vi "LP MDrive_Home.vi"(0 "VISA IN":refnum<visa-resource-name>="COM1", 1 "Home Direction":string="1", 5 "error in":errorcluster, 6 "Max Velocity to Home":string="1500", 9 "Mdrive Mode":T1=enum."Party Mode", 11 "Device Name":string="R", 12 "Timeout":u32=30000) -> (14 "VISA OUT":refnum<visa-resource-name>="COM1", 15 "Moved":bool, 19 "error out":errorcluster)   [LabVIEW 2015]
uses:
  MCode_LV_86/MDrive Mode.ctl
  MCode_LV_86/Set Parameter.ctl
  Stream/LP Globals.vi
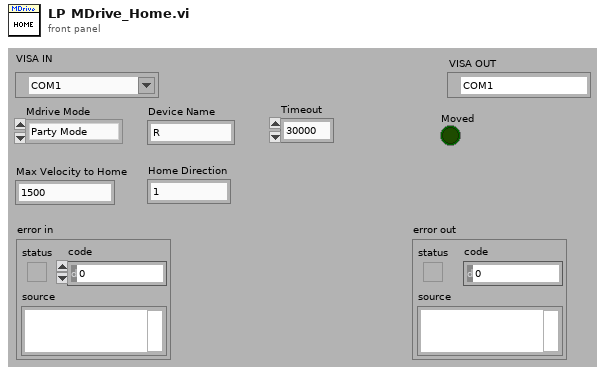
[diagram p1: front panel]
types:
  T1 = typedef "MDrive Mode.ctl" = enum16{"Normal Mode", "Party Mode"}
  T2 = typedef "Set Parameter.ctl" = enum16{"Acceleration (A)", "Baud Rate (BD)", "Counter 1 (C1)", "Counter 2 (C2)", "Control C Software Reset (CE)", "Check Sum Enable (CK)", "Clock Mode (CM)", "Clock Mode Ratio (CR)", "Clock Mode Out Step Width (CW)", "Deceleration (D)", "Digital Filtering, Input 1 (D1)", "Digital Filtering, Input 2 (D2)", "Digital Filtering, Input 3 (D3)", "Digital Filtering, Input 4 (D4)", "Digital Filtering, Input 5 (D5)", "Digital Filtering, Input 9 (D9)", "Digital Filtering, Input 10 (D10)", "Digital Filtering, Input 11 (D11)", "Digital Filtering, Input 12 (D12)", "Deadband (DB)", "Decrement Variable (DC)", "Enable/Disable Drive (DE)", "Device Name (DN)", "End Program Execution (E)", "Encoder Function Enable (EE)", "Encoder Lines (EL)", "Echo Mode (EM)", "Error Clear (ER)", "Escape (ES)", "Execute Program at Address (EX)", "Factory Default (FD)", "Hold (H)", "Hold Current (HC)", "Hold Current Encoder Index (HI)", "Home to Home Switch (HM)", "Home to Delay Time (HT)", "Increment Variable (IC)", "Initialize Parameters to NVM (IP)", "Input into Variable (IV)", "Jog Enable (JE)", "Limit Stop Mode (LM)", "Move Absolute (MA)", "Move Relative (MR)", "MicroStepping Select (MS)", "Motor Settling Delay Time (MT)", "Output 1 (O1)", "Output 2 (O2)", "Output 3 (O3)", "Output 4 (O4)", "Output 9 (O9)", "Output 10 (O10)", "Output 11 (O11)", "Output 12 (O12)", "Output High Byte (9-12) (OH)", "Output Low Byte (1-4) (OL)", "Output Total (1-4 and 9-12) (OT)", "Position (P)", "Position Maintenance (PM)", "Party Mode (PY)", "Register 1 (R1)", "Register 2 (R2)", "Register 3 (R3)", "Register 4 (R4)", "Run Current (RC)", "Stall Factor (SF)", "Slew (SL)", "Stall Mode Set (SM)", "Upgrade Firmware (UG)", "Velocity Initial (VI)", "Velocity Maximum (VM)", "Set Input #1 as Home (S1)", "Save (S)", "Save DN+PY (NameS)", "Active Party Mode (0x0A)", "Set Input #1 (S1) as Limit- Active Floating", "Set Input #2 (S2) as Limit+ Active Floating", "Set Input #1 as Home (S1) Active Floating", "Set Input #1 as Home (S2) Active Floating", "Set Input #1 (S1) as Limit+ Active Floating", "Set Input #2 (S2) as Limit- Active Floating", "Hybrid Mode (AS)"}
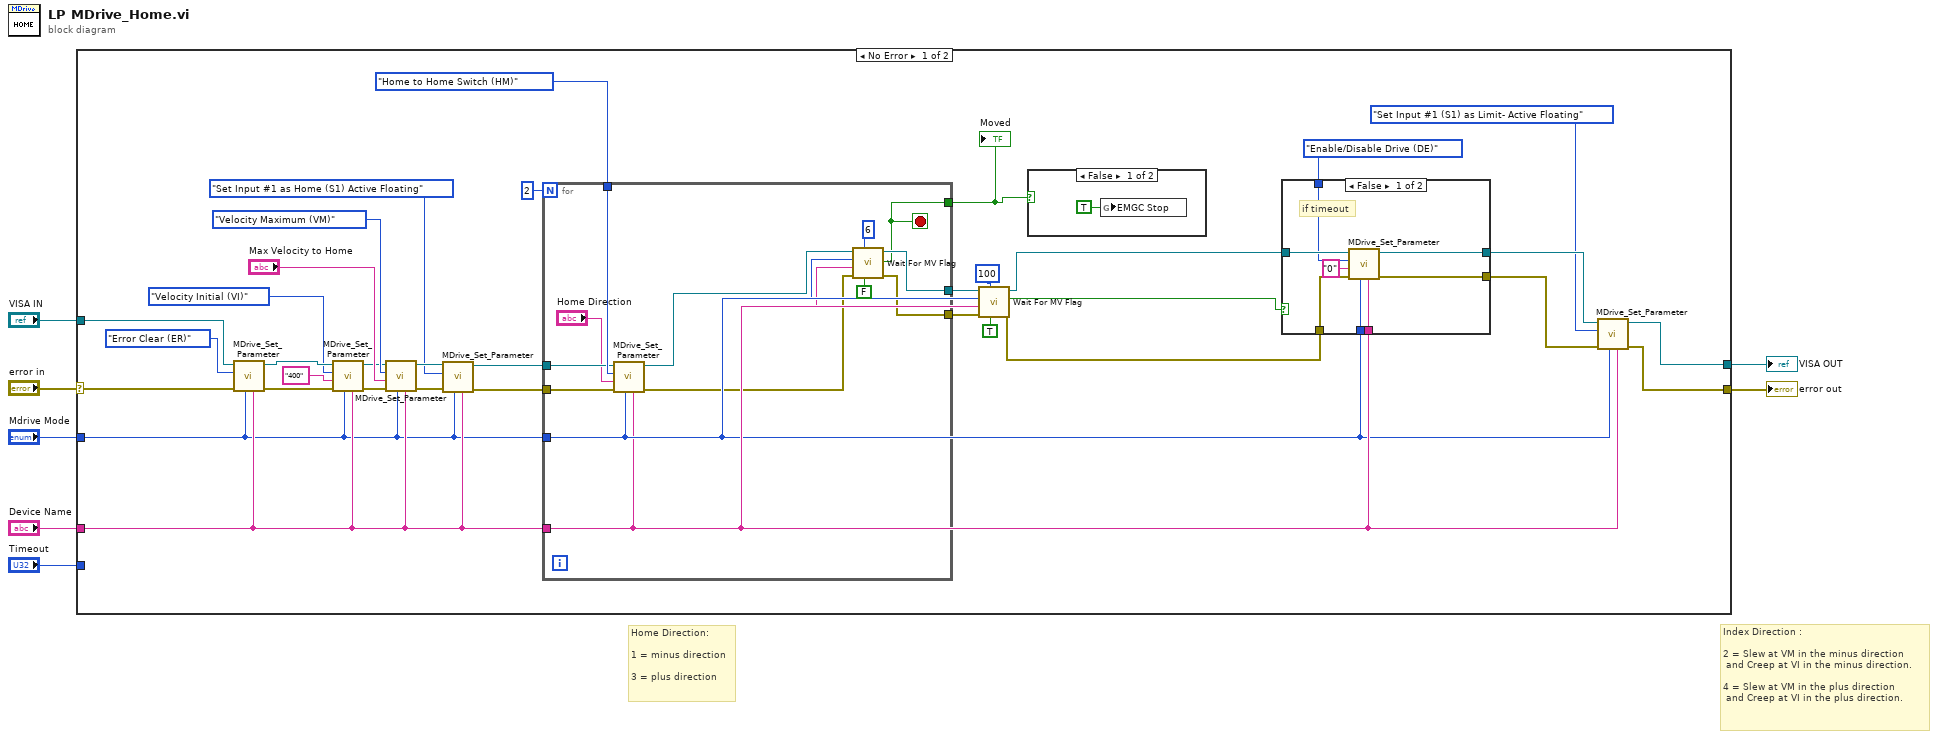
[diagram p0: block diagram]
diagram:
  # "Home Direction:\n\n1 = minus direction\n\n3 = plus direction"
  # "Index Direction :\n\n2 = Slew at VM in the minus direction\n and Creep at VI in the minus direction.\n\n4 = Slew at VM in the plus direction\n and Creep at VI in the plus direction."
  n1 = case shown="No Error" "error in" {
    selector: "error in" -> [w27 w67]
    tunnel: [w17 w66] -> w7
    tunnel: [w16 w67] -> w6
    tunnel: "VISA IN" -> [w35 w66]
    tunnel: "Timeout" -> [_ _]
    tunnel: "Mdrive Mode" -> [w10 _]
    tunnel: "Device Name" -> [w13 _]
    frame No Error {
      n2 = call "MDrive_Set_Parameter.vi"("Device Name"=w13, "Mdrive Mode"=w10, "error in"=w27, "Set Parameter"=Set_Parameter."Error Clear (ER)", "VISA IN"=w35) -> ("error out"=w38:errorcluster, "VISA OUT"=w37:refnum<visa-resource-name>)  [unwired: 4 in, 1 out]
      n3 = call "MDrive_Set_Parameter.vi"("Device Name"=w13, "Mdrive Mode"=w10, "error in"=w38, "Parameter Setpoint"="400", "Set Parameter"=Set_Parameter."Velocity Initial (VI)", "VISA IN"=w37) -> ("error out"=w36:errorcluster, "VISA OUT"=w34:refnum<visa-resource-name>)  [unwired: 3 in, 1 out]
      n4 = call "MDrive_Set_Parameter.vi"("Device Name"=w13, "Mdrive Mode"=w10, "error in"=w36, "Parameter Setpoint"="Max Velocity to Home", "Set Parameter"=Set_Parameter."Velocity Maximum (VM)", "VISA IN"=w34) -> ("error out"=w25:errorcluster, "VISA OUT"=w30:refnum<visa-resource-name>)  [unwired: 3 in, 1 out]
      n5 = call "MDrive_Set_Parameter.vi"("Device Name"=w13, "Mdrive Mode"=w10, "error in"=w25, "Set Parameter"=Set_Parameter."Set Input #1 as Home (S1) Active Floating", "VISA IN"=w30) -> ("error out"=w26:errorcluster, "VISA OUT"=w29:refnum<visa-resource-name>)  [unwired: 4 in, 1 out]
      n6 = for {
        N: 2 -> [_]
        tunnel: Set_Parameter."Home to Home Switch (HM)" ("Set Parameter") -> [w55]
        tunnel: w29 -> [w54]
        tunnel: w26 -> [w52]
        tunnel: w13 -> [w51]
        tunnel: [w49] -> w12
        tunnel: [w48] -> w11
        tunnel: w10 -> [w45]
        tunnel: [w43] -> w8
        stop <- w43 stop-if-true
        n7 = call "MDrive_Set_Parameter.vi"("Device Name"=w51, "Mdrive Mode"=w45, "error in"=w52, "Parameter Setpoint"="Home Direction", "Set Parameter"=w55, "VISA IN"=w54) -> ("error out"=w50:errorcluster, "VISA OUT"=w44:refnum<visa-resource-name>)  [unwired: 3 in, 1 out]
        n8 = call "Wait For MV Flag.vi"("WaitMode(T=Stop)"=FALSE, "Timeout(0.5S Cycles)"=6, "error in (no error)"=w50, "Device Name"=w51, "Mdrive Mode"=w45, "VISA Refnum in"=w44) -> ("error out"=w49:errorcluster, "OK"=w43:bool, "VISA Refnum out"=w48:refnum<visa-resource-name>)  [unwired: 3 in]
      }
      "Moved" <- w8
      n9 = call "Wait For MV Flag.vi"("WaitMode(T=Stop)"=TRUE, "Timeout(0.5S Cycles)"=100 ("Timeout(40mS Cycles)"), "error in (no error)"=w12, "Device Name"=w13, "Mdrive Mode"=w10, "VISA Refnum in"=w11) -> ("error out"=w22:errorcluster, "OK"=w24:bool, "VISA Refnum out"=w23:refnum<visa-resource-name>)  [unwired: 3 in]
      n10 = case shown="False" w8 {
        frame False {
          n11 = global write "LP Globals.vi" "EMGC Stop"(TRUE ("EMGC Stop")) -> ()
        }
        frame True {
        }
      }
      n12 = case shown="False" w24 {
        tunnel: w23 -> [w63 w64]
        tunnel: w22 -> [w62 w65]
        tunnel: w10 -> [w61 _]
        tunnel: w13 -> [w60 _]
        tunnel: Set_Parameter."Enable/Disable Drive (DE)" ("Set Parameter") -> [w59 _]
        tunnel: [w57 w64] -> w20
        tunnel: [w56 w65] -> w19
        frame False {
          # "if timeout"
          n13 = call "MDrive_Set_Parameter.vi"("Device Name"=w60, "Mdrive Mode"=w61, "error in"=w62, "Parameter Setpoint"="0", "Set Parameter"=w59, "VISA IN"=w63) -> ("error out"=w56:errorcluster, "VISA OUT"=w57:refnum<visa-resource-name>)  [unwired: 3 in, 1 out]
        }
        frame True {
        }
      }
      n14 = call "MDrive_Set_Parameter.vi"("Device Name"=w13, "Mdrive Mode"=w10, "error in"=w19, "Set Parameter"=Set_Parameter."Set Input #1 (S1) as Limit- Active Floating", "VISA IN"=w20) -> ("error out"=w16:errorcluster, "VISA OUT"=w17:refnum<visa-resource-name>)  [unwired: 4 in, 1 out]
    }
    frame Error {
    }
  }
  "VISA OUT" <- w7
  "error out" <- w6
